vi "QCA - DUT Start Rx.vi"(0 "CART TCP Connection In":refnum<k5>, 7 "Receive Config":T2={"Frequency, MHz"=2412, "Data Rate"="1,0,0", "Packet Count"=0, "RX Mac Address"="10:11:11:11:11:01", "TX Mac Address"="10:11:11:11:11:01", "BS Mac Address"="10:11:11:11:11:01", "Packet Length"=1000, "Broadcast"=FALSE}, 11 "error in (no error)":errorcluster) -> (4 "CART TCP Connection Out":refnum<k5>, 14 "Command Sent":string, 15 "error out":errorcluster)   [LabVIEW 2011]
uses:
  Controls/Data Rates.ctl
  Controls/Parameter.ctl
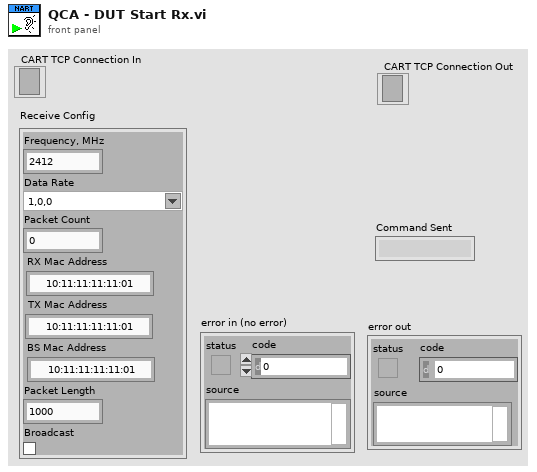
[diagram p1: front panel]
types:
  T1 = typedef "Data Rates.ctl" = string
  T2 = cluster{"Frequency, MHz":u32, "Data Rate":T1, "Packet Count":i32, "RX Mac Address":string, "TX Mac Address":string, "BS Mac Address":string, "Packet Length":u32, "Broadcast":bool}
  T3 = typedef "Parameter.ctl" = cluster{"Name":string, "Type":enum16{"decimal", "string", "float", "hex"}}
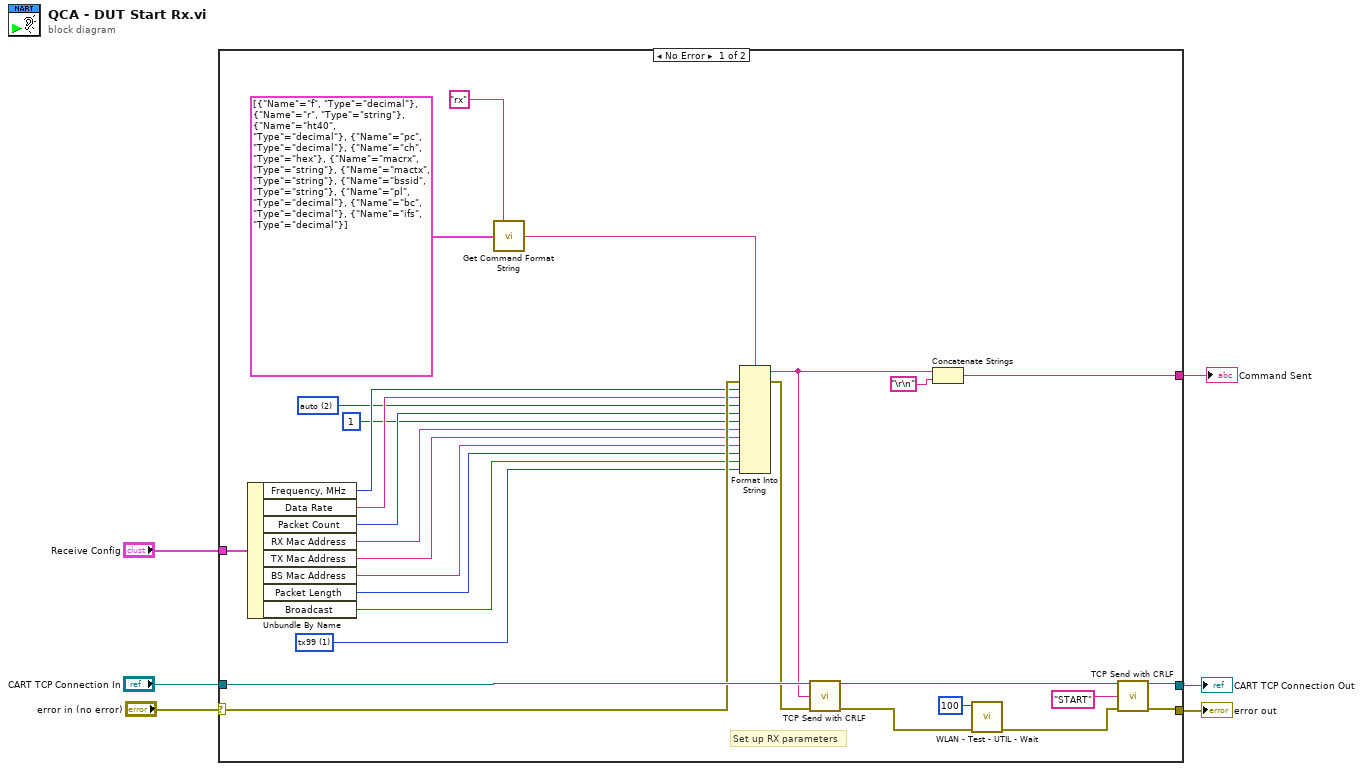
[diagram p0: block diagram]
diagram:
  n1 = case shown="No Error" "error in (no error)" {
    selector: "error in (no error)" -> [w31 w36]
    tunnel: [w26 w36] -> w5
    tunnel: "CART TCP Connection In" -> [w34 w35]
    tunnel: [w25 w35] -> w3
    tunnel: "Receive Config" -> [w29 _]
    tunnel: [w17 _] -> w1
    frame No Error {
      w10 = i16 1 items=["Regular"=-1, "tx100"=0, "tx99"=1] ("Inter Frame Spacing")
      w12 = i16 2 items=["none"=0, "low"=-1, "high"=1, "auto"=2] ("input 3")
      # "Set up RX parameters"
      n2 = Unbundle By Name(w29) -> ("Frequency, MHz"=w27:u32, "Data Rate"=w13:T1, "Packet Count"=w22:i32, "RX Mac Address"=w21:string, "TX Mac Address"=w20:string, "BS Mac Address"=w15:string, "Packet Length"=w19:u32, "Broadcast"=w14:bool)
      n3 = call "Get Command Format String.vi"("Command"="rx", "Parameters"=T3[] [{"Name"="f", "Type"=enum."decimal"}, {"Name"="r", "Type"=enum."string"}, {"Name"="ht40", "Type"=enum."decimal"}, {"Name"="pc", "Type"=enum."decimal"}, {"Name"="ch", "Type"=enum."hex"}, {"Name"="macrx", "Type"=enum."string"}, {"Name"="mactx", "Type"=enum."string"}, {"Name"="bssid", "Type"=enum."string"}, {"Name"="pl", "Type"=enum."decimal"}, {"Name"="bc", "Type"=enum."decimal"}, {"Name"="ifs", "Type"=enum."decimal"}]) -> ("Command Format String"=w28:string)  [unwired: 13 in]
      n4 = Format Into String(format string=w28, error in=w31, w27, w13, w12, w22, 1 ("Chains"), w21, w20, w15, w19, w14, w10) -> (resulting string=w16:string, error out=w30:errorcluster)  [unwired: 1 in]
      n5 = call "TCP Send with CRLF.vi"("CART TCP Connection"=w34, "data in"=w16, "error IO"=w30) -> ("CART TCP Connection Out"=w24:refnum<k5>, "error out"=w23:errorcluster)  [unwired: 11 in]
      n6 = Concatenate Strings(w16, "\r\n") -> (w17:string)
      n7 = call "WLAN - Test - UTIL - Wait.vi"("error in (no error)"=w23, "Wait (ms)"=u32 100) -> ("error out"=w9:errorcluster)  [unwired: 9 in]
      n8 = call "TCP Send with CRLF.vi"("CART TCP Connection"=w24, "data in"="START" ("format string"), "error IO"=w9) -> ("CART TCP Connection Out"=w25:refnum<k5>, "error out"=w26:errorcluster)  [unwired: 11 in]
    }
    frame Error {
    }
  }
  "error out" <- w5
  "CART TCP Connection Out" <- w3
  "Command Sent" <- w1
